vi "Moxom Run.vi"() -> ()   [LabVIEW 2011]
uses:
  <vilib>/Instr/_visa.llb/VISA Configure Serial Port (Instr).vi
panel:
  out "Kill Switch Enabled":bool
  in  "Durration":i32[](array[numeric])
  in  "Right Motor":i32[](array[numeric])
  in  "Left Motor":i32[](array[numeric])
  in  "Motor Controller\nSerial Port":refnum<visa-resource-name>
  out "Right Motor Remote":i32
  out "Right Motor Auto":i32
  out "Left Motor Remote":i32
  out "Left Motor Auto":i32
  out "Auto Enabled":bool
  in  "Auto":bool
  in  "stop":bool
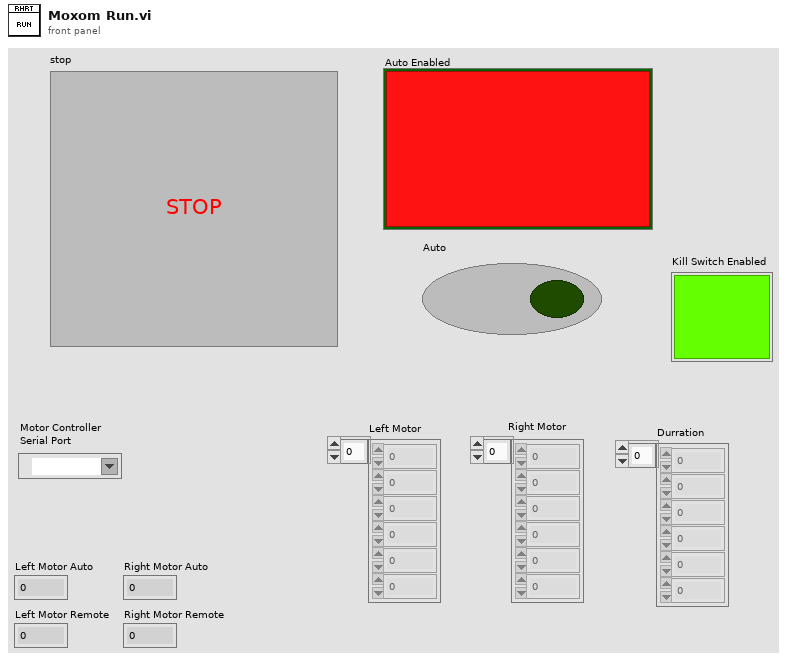
[diagram p1: front panel]
types:
  T1 = cluster{"axes total":u32, "buttons total":u32, "pov total":u32, "device name":string}[]
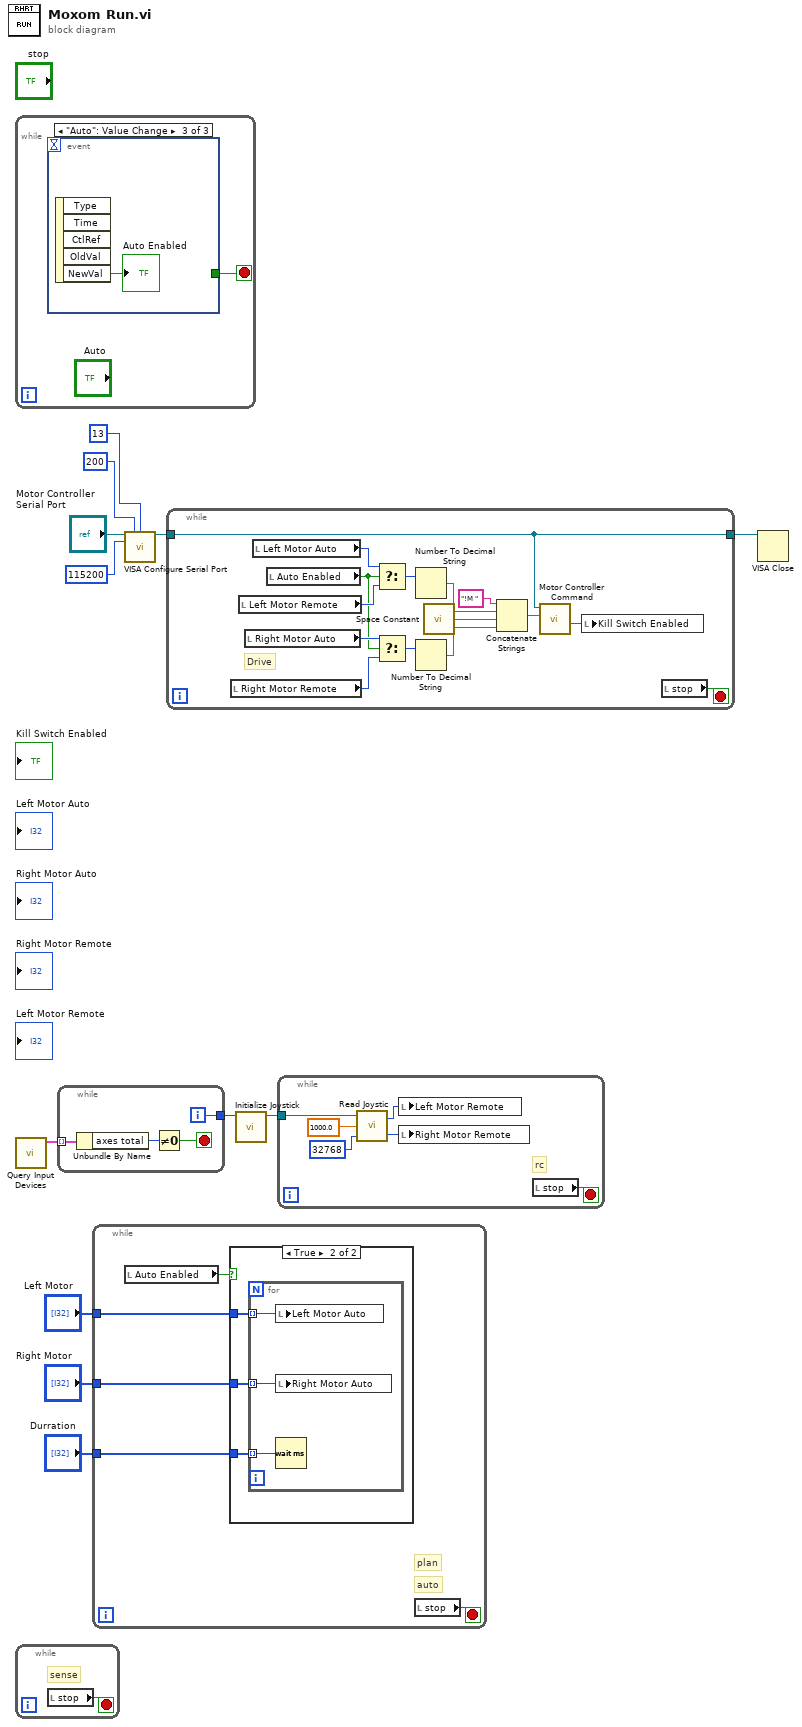
[diagram p0: block diagram]
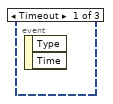
[diagram p3: hidden frame]
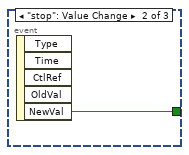
[diagram p4: hidden frame]
diagram:
  n1 = while {
    stop <- w13 stop-if-true
    n2 = event shown="[2] \"Auto\": Value Change" {
      selector: _ -> [_ _ _]
      dyn-events: _ -> [_ _ _]
      timeout: _ -> [_ _ _]
      tunnel: [_ w14 _] -> w13
      event Timeout {
        n3 = event-data() -> ()  [unwired: 1 in, 2 out]
      }
      event "stop": Value Change {
        n4 = event-data() -> ("NewVal"=w14:bool)  [unwired: 1 in, 4 out]
      }
      event "Auto": Value Change {
        n5 = event-data() -> ("NewVal"=→"Auto Enabled":bool)  [unwired: 1 in, 4 out]
      }
    }
  }
  n6 = call <vilib>:"Query Input Devices.vi"() -> ("joystick info"=w4:T1)  [unwired: 8 in, 3 out]
  n7 = while {
    stop <- w16 stop-if-true
    # "sense"
    n8 = local read "stop"() -> (w16:bool)
  }
  n9 = while {
    tunnel: w4 -> [w20] mode=indexing
    tunnel: [w17] -> w3
    i -> [w17]
    stop <- w18 stop-if-true
    n10 = Unbundle By Name(w20) -> ("axes total"=w19:u32)
    n11 = Not Equal To 0?(x=w19) -> (x != 0?=w18:bool)
  }
  n12 = while {
    tunnel: "Left Motor" -> [w23]
    tunnel: "Right Motor" -> [w22]
    tunnel: "Durration" -> [w21]
    stop <- w25 stop-if-true
    # "auto"
    # "plan"
    n13 = local read "Auto Enabled"() -> (w24:bool)
    n14 = case shown="True" w24 {
      tunnel: w23 -> [_ w28]
      tunnel: w22 -> [_ w27]
      tunnel: w21 -> [_ w26]
      frame False {
      }
      frame True {
        n15 = for {
          tunnel: w28 -> [w30] mode=indexing
          tunnel: w27 -> [w29] mode=indexing
          tunnel: w26 -> [w31] mode=indexing
          n16 = local write "Left Motor Auto"(w30) -> ()
          n17 = local write "Right Motor Auto"(w29) -> ()
          n18 = Wait (ms)(milliseconds to wait=w31) -> ()  [unwired: 1 out]
        }
      }
    }
    n19 = local read "stop"() -> (w25:bool)
  }
  n20 = call-poly "VISA Configure Serial Port"("VISA resource name"="Motor Controller\nSerial Port", "timeout (10sec)"=u32 200, "termination char\n(0xA = '\\n' = LF)"=u8 13 ("termination char\n(0xA = '\\n' = LF)"), "baud rate (9600)"=u32 115200) -> ("VISA resource name out"=w9:refnum<visa-resource-name>)  [unwired: 10 in, 1 out]
  n21 = while {
    tunnel: w9 -> [w36]
    tunnel: [w36] -> w8
    stop <- w46 stop-if-true
    # "Drive"
    n22 = local read "Right Motor Remote"() -> (w42:i32)
    n23 = local read "Left Motor Remote"() -> (w44:i32)
    n24 = local read "Right Motor Auto"() -> (w43:i32)
    n25 = local read "Left Motor Auto"() -> (w45:i32)
    n26 = local read "Auto Enabled"() -> (w41:bool)
    n27 = Select(t=w45, s=w41, f=w44) -> (s? t:f=w37:i32)
    n28 = Select(t=w43, s=w41, f=w42) -> (s? t:f=w38:i32)
    n29 = Number To Decimal String(number=w37) -> (decimal integer string=w34:string)  [unwired: 1 in]
    n30 = Number To Decimal String(number=w38) -> (decimal integer string=w33:string)  [unwired: 1 in]
    n31 = call <vilib>:"Space Constant.vi"() -> ("String"=w39:string)
    n32 = Concatenate Strings("!M " ("string"), w34, w39, w33) -> (w35:string)
    n33 = call "Motor Controller Command.vi"("Command"=w35, "VISA resource name"=w36) -> ("Timeout on read"=w32:bool)  [unwired: 6 in, 3 out]
    n34 = local write "Kill Switch Enabled"(w32) -> ()
    n35 = local read "stop"() -> (w46:bool)
  }
  n36 = call <vilib>:"Initialize Joystick.vi"("device index"=w3) -> ("device ID"=w2:refnum<k1>)  [unwired: 9 in, 1 out]
  n37 = while {
    tunnel: w2 -> [w47]
    stop <- w52 stop-if-true
    # "rc"
    n38 = call "Read Joystic.vi"("JoystickOutMaximum"=32768, "MaxMotorSpeed"=1000.0 ("HalfMaxMotorSpeed"), "device ID"=w47) -> ("Right Motor"=w48:i32, "Left Motor"=w49:i32)
    n39 = local write "Left Motor Remote"(w49) -> ()
    n40 = local write "Right Motor Remote"(w48) -> ()
    n41 = local read "stop"() -> (w52:bool)
  }
  n42 = VISA Close(VISA resource name=w8) -> ()  [unwired: 1 in, 1 out]
